vi "Bemerkung Array Size.vi"(8 "error in":errorcluster, 9 "Bemerkungen (Eingang)":T9[](array[typedef]) {"Align (Left)" items=["Center", "Justified", "Justified All", "Left", "Right"]}, 10 "Table Array (Eingang)":T1[](array[typedef]) {"Horizontal Align" items=["Center", "Justified", "JustifiedAll", "Left", "Right"]; "TablePictures"."Horizontal Align" items=["Center", "Justified", "JustifiedAll", "Left", "Right"]; "Results"."Position" items=["First", "Last"]; "Results"."Horizontal Align" items=["Center", "Justified", "JustifiedAll", "Left", "Right"]}, 11 "Graph Array (Eingang)":T7[](array[typedef]) {"Align (Left)" items=["Center", "Justified", "Justified All", "Left", "Right"]}) -> (0 "error out":errorcluster, 1 "Bemerkungen (Ausgang)":T9[](array[typedef]) {"Align (Left)" items=["Center", "Justified", "Justified All", "Left", "Right"]}, 2 "Table Array (Ausgang)":T1[](array[typedef]) {"Horizontal Align" items=["Center", "Justified", "JustifiedAll", "Left", "Right"]; "TablePictures"."Horizontal Align" items=["Center", "Justified", "JustifiedAll", "Left", "Right"]; "Results"."Position" items=["First", "Last"]; "Results"."Horizontal Align" items=["Center", "Justified", "JustifiedAll", "Left", "Right"]}, 3 "Graph Array (Ausgang)":T7[](array[typedef]) {"Align (Left)" items=["Center", "Justified", "Justified All", "Left", "Right"]})   [LabVIEW 2020, in "PDF Interface.lvlib" / "PDF Interface Helper.lvlib"]
uses:
  PDF Interface Helper.lvlib
  PDFBemerkung.ctl
  <vilib>/Simplicity AI/SAI_PDF_API/Classes/Context/Controls/SAI_PDF_Text Align.ctl
  <vilib>/Simplicity AI/SAI_PDF_API/Classes/Context/Controls/SAI_PDF_Font.ctl
  <vilib>/Simplicity AI/SAI_PDF_API/Classes/Context/Controls/SAI_PDF_Font Encoding.ctl
  PDFTableContentType.ctl
  PDFResults.ctl
  PDFResultPictures.ctl
  PDFCommentPosition.ctl
  PDFPageBreak.ctl
  PDFTablePictures.ctl
  PDFGraph.ctl
  <vilib>/Simplicity AI/SAI_PDF_API/Classes/Context/Context.lvclass
panel:
  # "(Cp1252)"
  # "(Cp1252)"
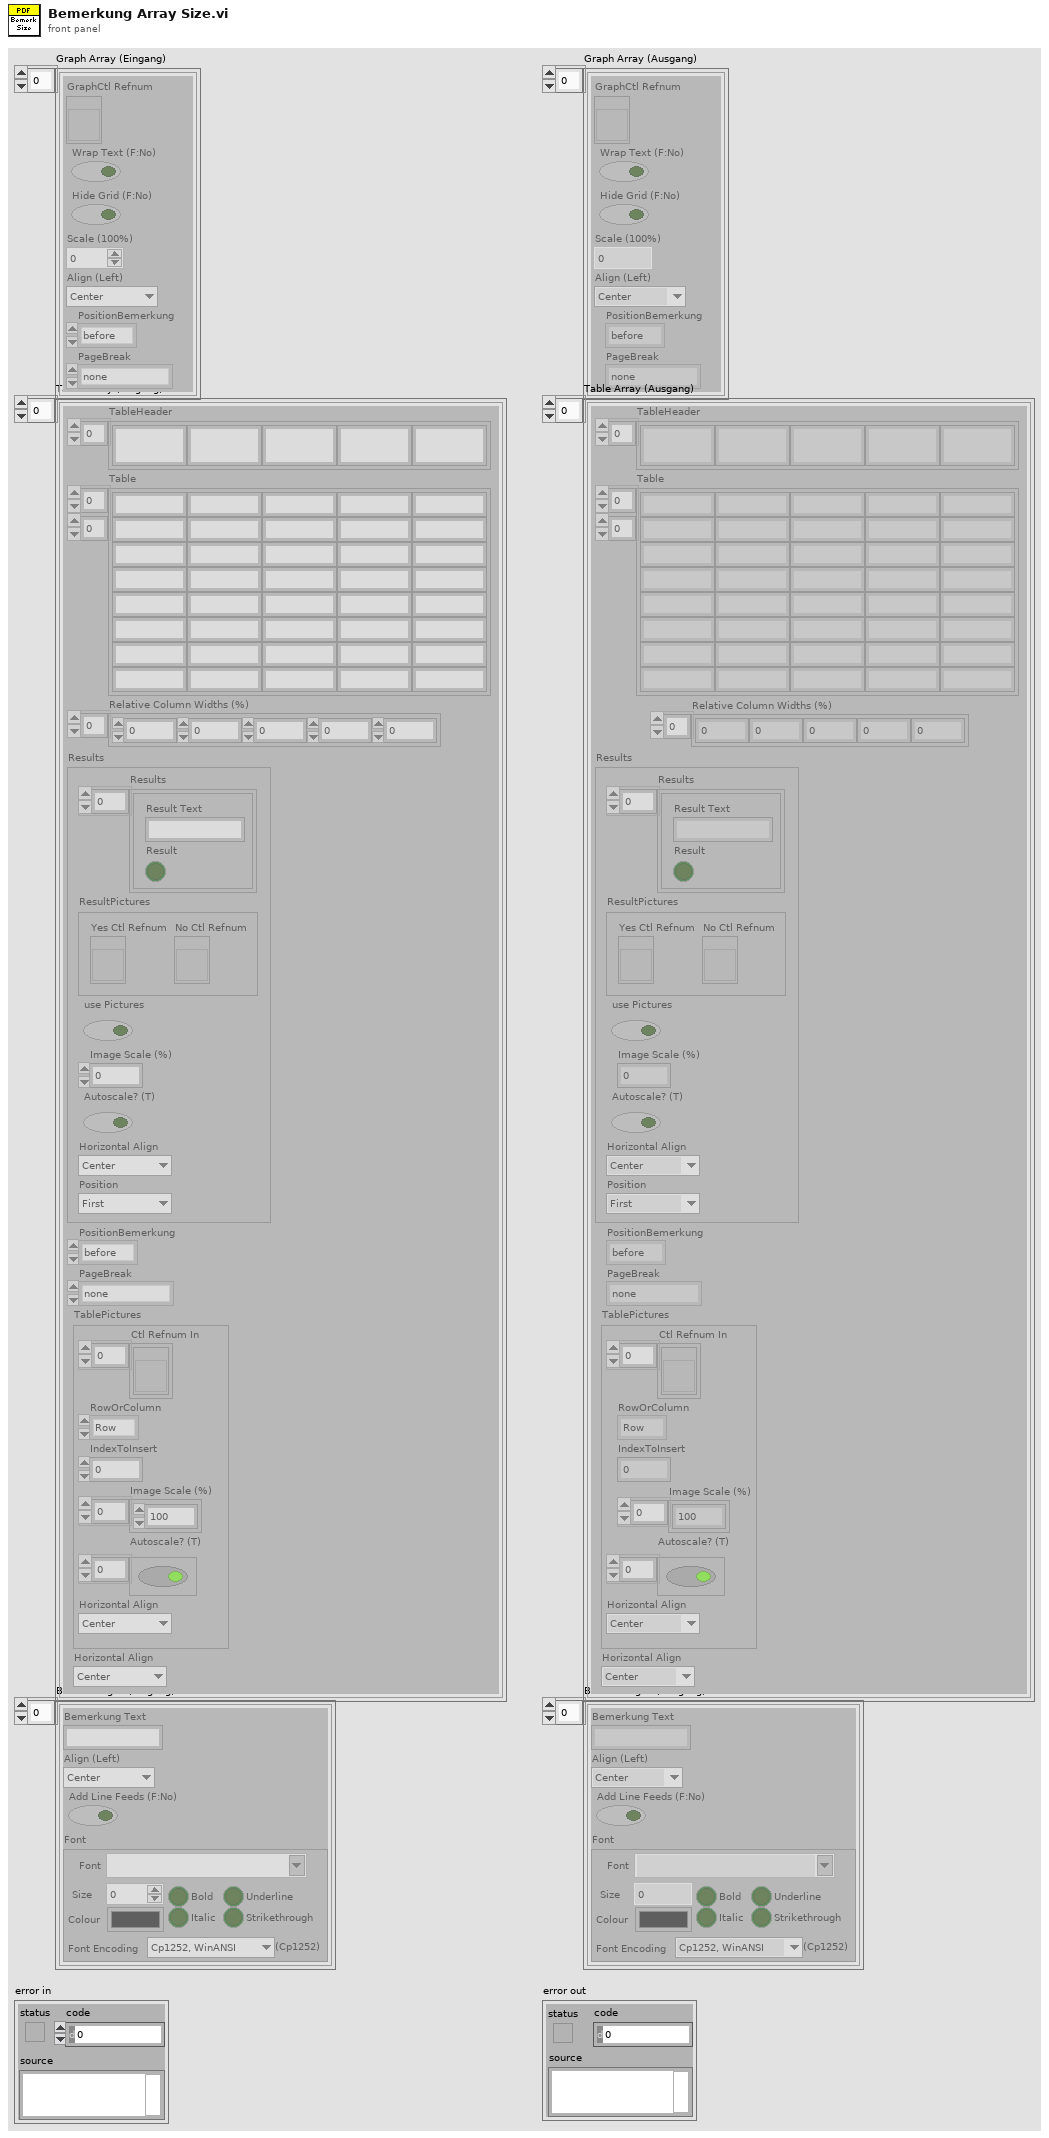
[diagram p1: front panel]
types:
  T1 = typedef "PDF Interface.lvlib/PDF Interface Helper.lvlib/PDFTableContentType.ctl" = cluster{"TableHeader":string[], "Table":string[][], "Relative Column Widths (%)":sgl[], "Results":T2, "PositionBemerkung":T4, "PageBreak":T5, "TablePictures":T6, "Horizontal Align":i32}
  T2 = typedef "PDF Interface.lvlib/PDF Interface Helper.lvlib/PDFResults.ctl" = cluster{"Results":cluster{"Result Text":string, "Result":bool}[], "ResultPictures":T3, "use Pictures":bool, "Image Scale (%)":sgl, "Autoscale? (T)":bool, "Horizontal Align":i32, "Position":i32}
  T3 = typedef "PDF Interface.lvlib/PDF Interface Helper.lvlib/PDFResultPictures.ctl" = cluster{"Yes Ctl Refnum":refnum<vi>, "No Ctl Refnum":refnum<vi>}
  T4 = typedef "PDF Interface.lvlib/PDF Interface Helper.lvlib/PDFCommentPosition.ctl" = enum16{"before", "after"}
  T5 = typedef "PDF Interface.lvlib/PDF Interface Helper.lvlib/PDFPageBreak.ctl" = enum16{"none", "before", "after", "after comment"}
  T6 = typedef "PDF Interface.lvlib/PDF Interface Helper.lvlib/PDFTablePictures.ctl" = cluster{"Ctl Refnum In":refnum<vi>[], "RowOrColumn":enum16{"Row", "Column"}, "IndexToInsert":u16, "Image Scale (%)":sgl[], "Autoscale? (T)":bool[], "Horizontal Align":i32}
  T7 = typedef "PDF Interface.lvlib/PDF Interface Helper.lvlib/PDFGraph.ctl" = cluster{"GraphCtl Refnum":refnum<vi>, "Wrap Text (F:No)":bool, "Hide Grid (F:No)":bool, "Scale (100%)":sgl, "Align (Left)":T8, "PositionBemerkung":T4, "PageBreak":T5}
  T8 = typedef "SAI_PDF_Toolkit.lvlib/Context.lvclass/SAI_PDF_Text Align.ctl" = i32
  T9 = typedef "PDF Interface.lvlib/PDF Interface Helper.lvlib/PDFBemerkung.ctl" = cluster{"Bemerkung Text":string, "Align (Left)":T8, "Add Line Feeds (F:No)":bool, "Font":T10}
  T10 = typedef "SAI_PDF_Toolkit.lvlib/Context.lvclass/SAI_PDF_Font.ctl" = cluster{"Font":string, "Size":i32, "Colour":u32, "Bold":bool, "Italic":bool, "Underline":bool, "Strikethrough":bool, "Font Encoding":T11}
  T11 = typedef "SAI_PDF_Toolkit.lvlib/Context.lvclass/SAI_PDF_Font Encoding.ctl" = enum16{"Cp1252, WinANSI", "IdentityH", "IdentityV", "Cp1250", "Cp1257", "MacRoman"}
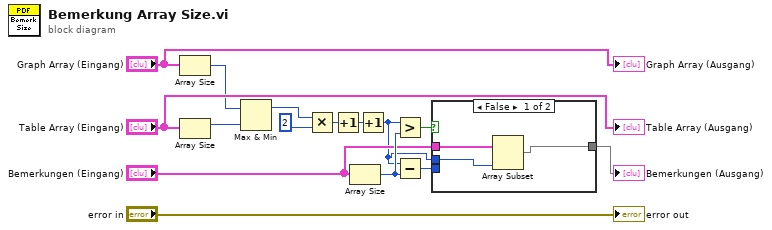
[diagram p0: block diagram]
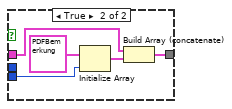
[diagram p2: hidden frame]
diagram:
  n1 = Array Size(array="Graph Array (Eingang)") -> (size(s)=w5:i32)
  n2 = Array Size(array="Table Array (Eingang)") -> (size(s)=w4:i32)
  n3 = Max & Min(x=w5, y=w4) -> (max(x,y)=w3:i32)  [unwired: 1 out]
  n4 = Multiply(x=w3, y=2) -> (x*y=w1:i32)
  n5 = Increment(x=w1) -> (x+1=w10:i32)
  n6 = Array Size(array="Bemerkungen (Eingang)") -> (size(s)=w13:i32)
  n7 = Increment(x=w10) -> (x+1=w6:i32)
  n8 = Greater?(x=w6, y=w13) -> (0:w11:bool)
  n9 = Subtract(x=w6, y=w13) -> (x-y=w14:i32)
  n10 = case shown="False" w11 {
    tunnel: "Bemerkungen (Eingang)" -> [w18 w22]
    tunnel: w14 -> [_ w23]
    tunnel: [w17 w20] -> w15
    tunnel: w6 -> [w16 _]
    frame False {
      n11 = Array Subset(array=w18, length=w16) -> (w17:T9[])  [unwired: 1 in]
    }
    frame True {
      n12 = Initialize Array(T9 {"Bemerkung Text"="", "Align (Left)"=0, "Add Line Feeds (F:No)"=FALSE, "Font"={"Font"="Arial", "Size"=10, "Colour"=0, "Bold"=FALSE, "Italic"=FALSE, "Underline"=FALSE, "Strikethrough"=FALSE, "Font Encoding"=enum."Cp1252, WinANSI"}} ("Bemerkung"), w23) -> (w21:T9[])
      n13 = Build Array (concatenate)(w22, w21) -> (w20:T9[])
    }
  }
  "Bemerkungen (Ausgang)" <- w15
  "Graph Array (Ausgang)" <- "Graph Array (Eingang)"
  "Table Array (Ausgang)" <- "Table Array (Eingang)"
  "error out" <- "error in"
